vi "ma_Compute H(w) from h(n).vi"(0 "h":dbl[](array[numeric]) format="%0.2f", 1 "FFT size":i32=1024) -> (2 "Mag H(w)":dbl[](array[numeric]) format="%0.2f", 3 "Phase H(w)":dbl[](array[numeric]) format="%0.2f", 4 "df":dbl format="%0.2f")   [LabVIEW 2020, in "NI_MAPro.lvlib"]
uses:
  NI_MAPro.lvlib
  NI_AALPro.lvlib
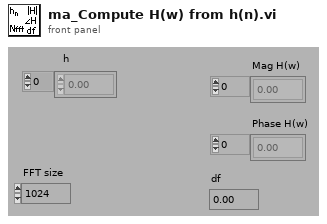
[diagram p1: front panel]
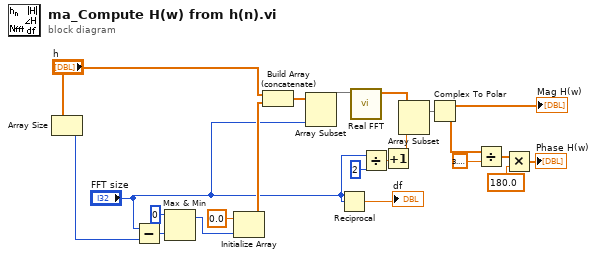
[diagram p0: block diagram]
diagram:
  n1 = Array Size(array="h") -> (size(s)=w16:i32)
  n2 = Subtract(x="FFT size", y=w16) -> (x-y=w11:i32)
  n3 = Max & Min(x=0, y=w11) -> (max(x,y)=w9:i32)  [unwired: 1 out]
  n4 = Initialize Array(0.0, w9) -> (w15:dbl[])
  n5 = Build Array (concatenate)("h", w15) -> (w8:dbl[])
  n6 = Array Subset(array=w8, length="FFT size") -> (w7:dbl[])  [unwired: 1 in]
  n7 = Reciprocal(x="FFT size") -> (1/x=→"df":dbl)
  n8 = call "Real FFT.vi"("X"=w7) -> ("FFT {X}"=w14:cdb[])  [unwired: 9 in, 1 out]
  n9 = Divide(x="FFT size", y=2) -> (x/y=w21:dbl)
  n10 = Increment(x=w21) -> (x+1=w20:dbl)
  n11 = Array Subset(array=w14, length=w20) -> (w13:cdb[])  [unwired: 1 in]
  n12 = Complex To Polar(r * e^(i*theta)=w13) -> (r=→"Mag H(w)":dbl[], theta=w2:dbl[])
  n13 = Divide(x=w2, y=3.141592653589793) -> (x/y=w4:dbl[])
  n14 = Multiply(x=w4, y=180.0) -> (x*y=→"Phase H(w)":dbl[])
